vi "lire code de LabelShop.vi"() -> ()   [LabVIEW 2011]
uses:
  <vilib>/Instr/_visa.llb/VISA Configure Serial Port (Instr).vi
panel:
  in  "nb d'octets à lire":u32=10000
  in  "delay before read (ms)":u32=500 caption="attente avant lecture (ms)"
  in  "flow control":u16(ring) caption="contrôle du flux" items=["Aucune"=0, "XON/XOFF"=1, "RTS/CTS"=2, "DTR/DSR"=4]
  in  "stop bits":u16(ring)=10 caption="bits de stop" items=["1.0"=10, "1.5"=15, "2.0"=20]
  in  "write":bool caption="écriture"
  in  "string to write":string caption="chaîne à écrire"
  in  "read":bool=TRUE caption="lire"
  out "bytes read":u32 caption="octets lus"
  out "read string":string caption="chaîne lue"
  in  "parity":u16(ring) caption="parité" items=["Aucune", "Impaire", "Paire", "Marque", "Espace"]
  in  "data bits":u16=8 caption="bits de données" min=5 max=8 step=1
  in  "baud rate":u32=9600 caption="débit en bauds"
  in  "VISA resource name":refnum<visa-resource-name>="COM3" caption="Nom de ressource VISA"
  # "- Relier les ports COM4 et COM3 du PC\n- Lancer le VI et lancer immédiatement une impression avec le logiciel LabelShop (s'assurer que   l'imprimante Easycoder PC4 est bien configurée en port COM4).\n- Récupérer le code émis par le logiciel pour pouvoir l'utiliser avec Labview."
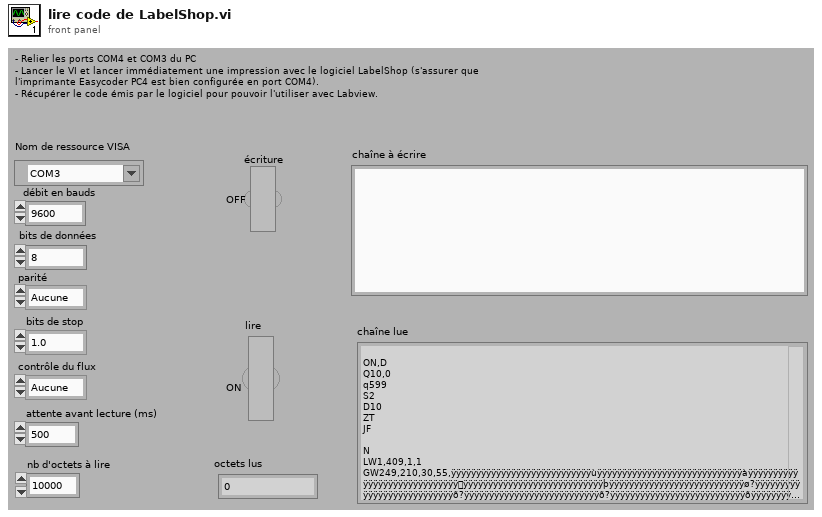
[diagram p1: front panel]
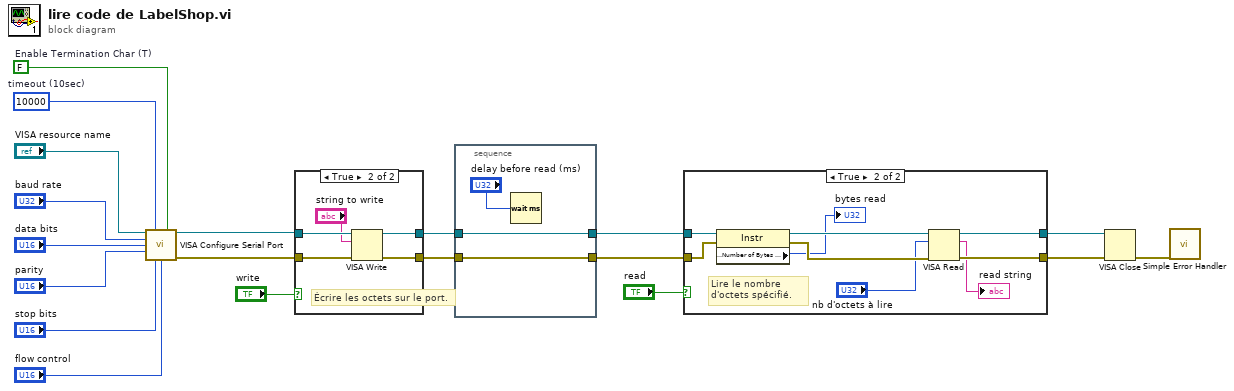
[diagram p0: block diagram]
diagram:
  w14 = FALSE  # Enable Termination Char (T)
  w15 = u32 10000  # timeout (10sec)
  n1 = call-poly "VISA Configure Serial Port"("VISA resource name"="VISA resource name", "timeout (10sec)"=w15, "Enable Termination\nChar (T)"=w14, "baud rate (9600)"="baud rate", "data bits (8)"="data bits", "parity (0:none)"="parity", "stop bits (10: 1 bit)"="stop bits", "flow control (0:none)"="flow control") -> ("VISA resource name out"=w9:refnum<visa-resource-name>, "error out"=w11:errorcluster)  [unwired: 6 in]
  n2 = case shown="True" "write" {
    tunnel: [w21 w26] -> w8
    tunnel: w9 -> [w20 w25]
    tunnel: w11 -> [w21 w24]
    tunnel: [w20 w23] -> w7
    frame False {
    }
    frame True {
      # "Écrire les octets sur le port."
      n3 = VISA Write(VISA resource name=w25, write buffer="string to write", error in (no error)=w24) -> (VISA resource name out=w23:refnum<visa-resource-name>, error out=w26:errorcluster)  [unwired: 1 out]
    }
  }
  n4 = stacked-sequence {
    tunnel: w8 -> [w29]
    tunnel: [w29] -> w6
    tunnel: w7 -> [w28]
    tunnel: [w28] -> w5
    frame #0 {
      n5 = Wait (ms)(milliseconds to wait="delay before read (ms)") -> ()  [unwired: 1 out]
    }
  }
  n6 = case shown="True" "read" {
    tunnel: w6 -> [w31 w36]
    tunnel: [w31 w40] -> w2
    tunnel: [w30 w39] -> w1
    tunnel: w5 -> [w30 w38]
    frame False {
    }
    frame True {
      # "Lire le nombre d'octets spécifié."
      n7 = property class="Instr"(reference=w38, error in=w36) -> (reference out=w37:refnum<visa-resource-name>, error out=w35:errorcluster, "Serial Settings:Number of Bytes at Serial Port"=→"bytes read":u32)
      n8 = VISA Read(VISA resource name=w37, byte count="nb d'octets à lire", error in (no error)=w35) -> (VISA resource name out=w39:refnum<visa-resource-name>, read buffer=→"read string":string, error out=w40:errorcluster)  [unwired: 1 out]
    }
  }
  n9 = VISA Close(VISA resource name=w1, error in (no error)=w2) -> (error out=w3:errorcluster)
  n10 = call <vilib>:"Simple Error Handler.vi"("error in (no error)"=w3) -> ()  [unwired: 4 in, 5 out]
